vi "Set Alias.vi"(6 "Previous Alias":string, 8 "error in (no error)":errorcluster, 9 "Endpoint":string, 10 "Alias":string, 11 "Aliases Ref in":T1 format="%.0x") -> (0 "error out":errorcluster, 3 "Aliases Ref out":T1 format="%.0x")   [LabVIEW 2020, in "Routing and Faulting System Explorer.lvlib"]
uses:
  Routing and Faulting System Explorer.lvlib
  <vilib>/NI VeriStand/Custom Device API/Custom Device Item Ref.ctl
  Parse Endpoint.vi
  Scripting/Routing and Faulting Scripting.lvlib
  <vilib>/NI VeriStand/Custom Device API/Custom Device API.lvlib
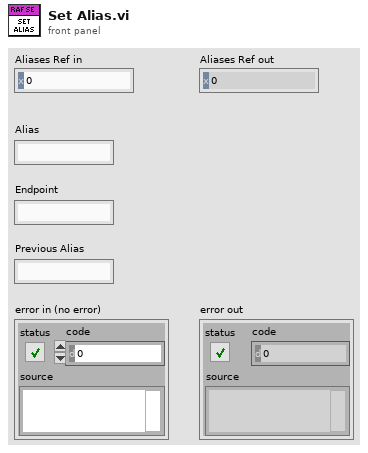
[diagram p1: front panel]
types:
  T1 = typedef "Custom Device API.lvlib/Custom Device Item Ref.ctl" = u64
  T2 = typedef "Routing and Faulting Shared.lvlib/Alias Endpoint.ctl" = cluster{"Module Path":string, "Endpoint":string}
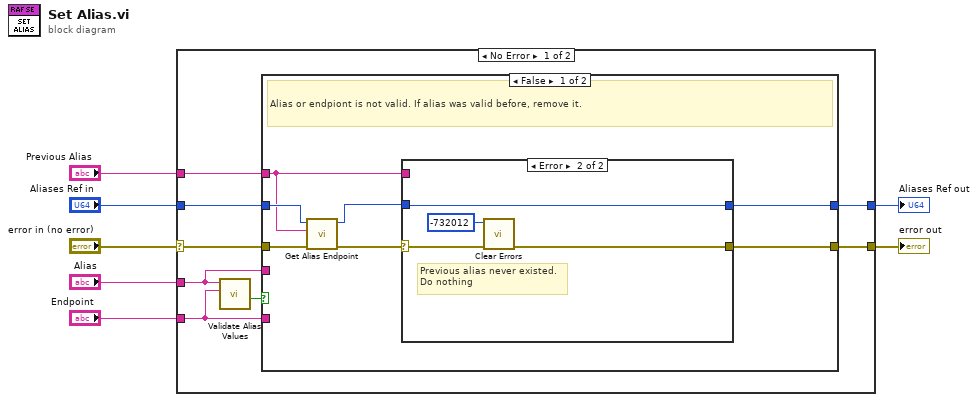
[diagram p0: block diagram]
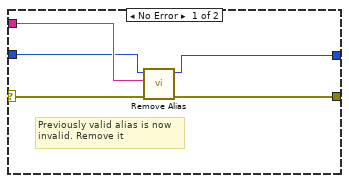
[diagram p2: hidden frame]
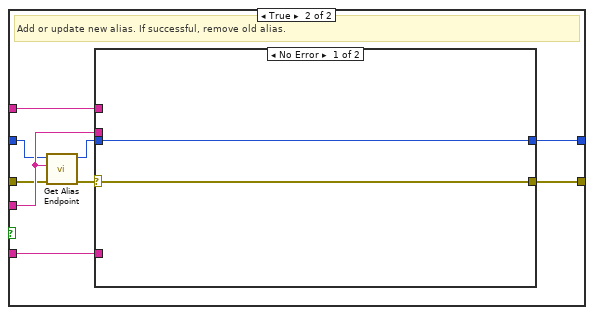
[diagram p3: hidden frame]
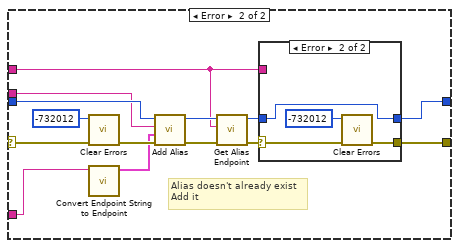
[diagram p4: hidden frame]
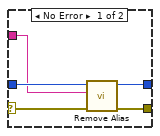
[diagram p5: hidden frame]
diagram:
  n1 = case shown="No Error" "error in (no error)" {
    selector: "error in (no error)" -> [w8 w66]
    tunnel: "Aliases Ref in" -> [w15 w67]
    tunnel: [w14 w66] -> w6
    tunnel: [w13 w67] -> w5
    tunnel: "Alias" -> [w12 _]
    tunnel: "Previous Alias" -> [w10 _]
    tunnel: "Endpoint" -> [w9 _]
    frame No Error {
      n2 = call "Validate Alias Values.vi"("Endpoint"=w9, "Alias"=w12) -> ("Valid"=w11:bool)  [unwired: 8 in, 1 out]
      n3 = case shown="False" w11 {
        tunnel: w12 -> [_ w38]
        tunnel: w15 -> [w21 w33]
        tunnel: w8 -> [w22 w36]
        tunnel: [w17 w35] -> w14
        tunnel: [w18 w34] -> w13
        tunnel: w10 -> [w16 w32]
        tunnel: w9 -> [_ w37]
        frame False {
          # "Alias or endpiont is not valid. If alias was valid before, remove it."
          n4 = call "Get Alias Endpoint.vi"("error in"=w22, "alias"=w16, "endpoint aliases in"=w21) -> ("error out"=w20:errorcluster, "endpoint aliases out"=w19:T1)  [unwired: 6 in, 1 out]
          n5 = case shown="Error" w20 {
            selector: w20 -> [w27 w30]
            tunnel: w19 -> [w23 w31]
            tunnel: [w26 w31] -> w18
            tunnel: [w24 w28] -> w17
            tunnel: w16 -> [w25 _]
            frame No Error {
              # "Previously valid alias is now\ninvalid. Remove it"
              n6 = call "Remove Alias.vi"("error in"=w27, "alias"=w25, "endpoint aliases in"=w23) -> ("error out"=w24:errorcluster, "endpoint aliases out"=w26:T1)  [unwired: 7 in]
            }
            frame Error {
              # "Previous alias never existed.\nDo nothing"
              n7 = call <vilib>:"Clear Errors.vi"("error in (no error)"=w30, "specific error code to clear (0: all)"=-732012) -> ("error out"=w28:errorcluster)  [unwired: 4 in, 1 out]
            }
          }
        }
        frame True {
          # "Add or update new alias. If successful, remove old alias."
          n8 = call "Get Alias Endpoint.vi"("error in"=w36, "alias"=w38, "endpoint aliases in"=w33) -> ("error out"=w40:errorcluster, "endpoint aliases out"=w39:T1)  [unwired: 6 in, 1 out]
          n9 = case shown="No Error" w40 {
            selector: w40 -> [w41 w47]
            tunnel: w39 -> [w42 w56]
            tunnel: w37 -> [_ w44]
            tunnel: w38 -> [_ w55]
            tunnel: [w41 w49] -> w35
            tunnel: [w42 w48] -> w34
            tunnel: w32 -> [_ w50]
            frame No Error {
            }
            frame Error {
              # "Alias doesn't already exist\nAdd it"
              n10 = call <vilib>:"Clear Errors.vi"("error in (no error)"=w47, "specific error code to clear (0: all)"=-732012) -> ("error out"=w46:errorcluster)  [unwired: 4 in, 1 out]
              n11 = call "Convert Endpoint String to Endpoint.vi"("Endpoint String"=w44) -> ("Endpoint"=w43:T2)  [unwired: 10 in]
              n12 = call "Add Alias.vi"("error in"=w46, "endpoint"=w43, "alias"=w55, "endpoint aliases in"=w56) -> ("error out"=w52:errorcluster, "endpoint aliases out"=w51:T1)  [unwired: 6 in]
              n13 = call "Get Alias Endpoint.vi"("error in"=w52, "alias"=w50, "endpoint aliases in"=w51) -> ("error out"=w54:errorcluster, "endpoint aliases out"=w53:T1)  [unwired: 6 in, 1 out]
              n14 = case shown="Error" w54 {
                selector: w54 -> [w61 w65]
                tunnel: w53 -> [w60 w62]
                tunnel: w50 -> [w59 _]
                tunnel: [w58 w63] -> w49
                tunnel: [w57 w62] -> w48
                frame No Error {
                  n15 = call "Remove Alias.vi"("error in"=w61, "alias"=w59, "endpoint aliases in"=w60) -> ("error out"=w58:errorcluster, "endpoint aliases out"=w57:T1)  [unwired: 7 in]
                }
                frame Error {
                  n16 = call <vilib>:"Clear Errors.vi"("error in (no error)"=w65, "specific error code to clear (0: all)"=-732012) -> ("error out"=w63:errorcluster)  [unwired: 4 in, 1 out]
                }
              }
            }
          }
        }
      }
    }
    frame Error {
    }
  }
  "Aliases Ref out" <- w5
  "error out" <- w6
